vi "DAQ 다지털 실습 종합.vi"() -> ()   [LabVIEW 2020]
uses:
  <vilib>/DAQmx/read.llb/DAQmx Read (Digital 1D Bool 1Chan 1Samp).vi
  <vilib>/DAQmx/write.llb/DAQmx Write (Digital 1D Bool 1Chan 1Samp).vi
  <vilib>/DAQmx/create/channels.llb/DAQmx Create Channel (DO-Digital Output).vi
  <vilib>/DAQmx/create/channels.llb/DAQmx Create Channel (DI-Digital Input).vi
  <vilib>/DAQmx/miscellaneous.llb/DAQmx Fill In Error Info.vi
  <vilib>/DAQmx/read.llb/DAQmx Read (Digital 1D Bool NChan 1Samp 1Line).vi
panel:
  in  "정지":bool
  out "data":bool[](array[boolean]) caption="데이터"
  in  "배열":bool[](array[boolean])
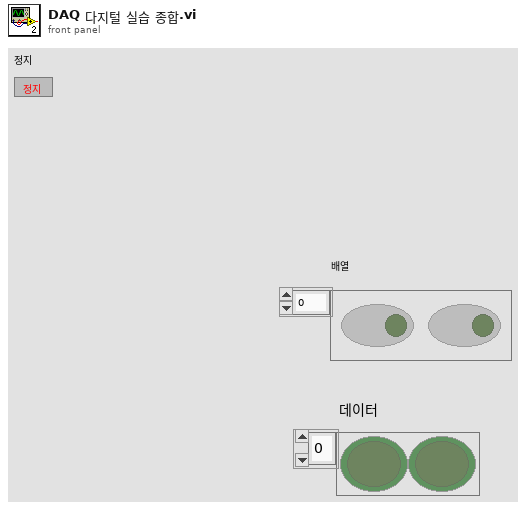
[diagram p1: front panel]
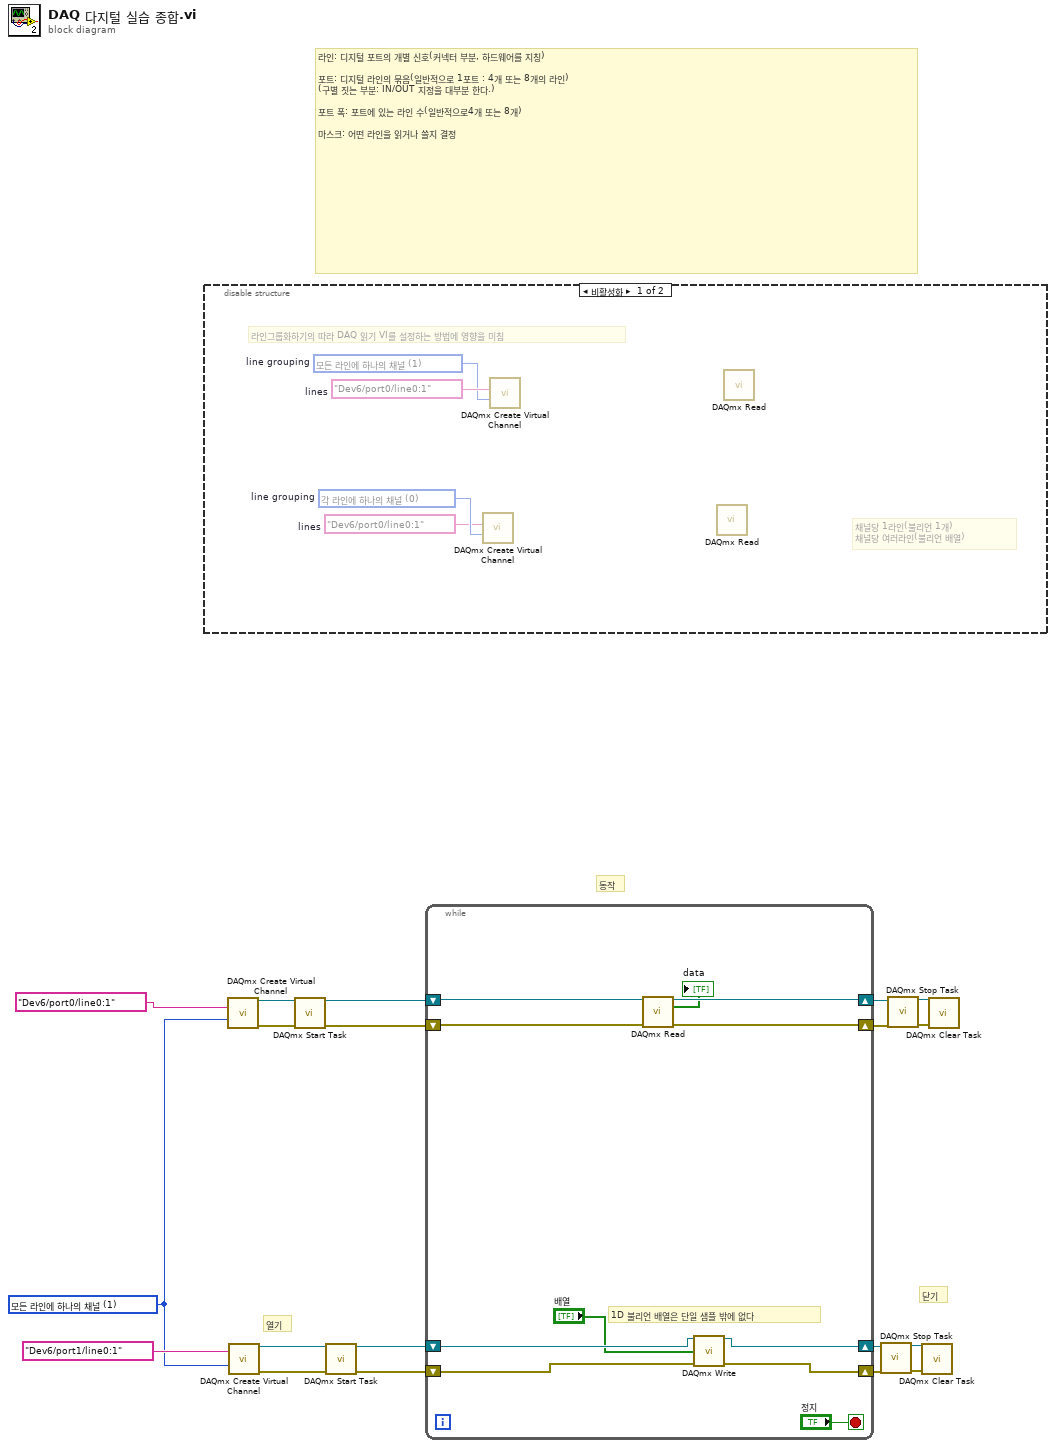
[diagram p0: block diagram]
diagram:
  w7 = 1 items=["각 라인에 하나의 채널", "모든 라인에 하나의 채널"] ("line grouping")
  # "닫기"
  # "동작"
  # "열기"
  # "라인: 디지털 포트의 개별 신호(커넥터 부분, 하드웨어를 지칭)\n\n포트: 디지털 라인의 묶음(일반적으로 1포트 : 4개 또는 8개의 라인)\n(구별 짓는 부분: IN/OUT 지정을 대부분 한다.)\n\n포트 폭: 포트에 있는 라인 수(일반적으로4개 또는 8개)\n\n마스크: 어떤 라인을 읽거나 쓸지 결정"
  n1 = disable-structure shown="비활성화" {
    frame Disabled {
      w21 = 0 items=["각 라인에 하나의 채널", "모든 라인에 하나의 채널"]  # line grouping
      w20 = tag "Dev6/port0/line0:1"  # lines
      w22 = 1 items=["각 라인에 하나의 채널", "모든 라인에 하나의 채널"]  # line grouping
      w23 = tag "Dev6/port0/line0:1"  # lines
      # "채널당 1라인(불리언 1개)\n채널당 여러라인(불리언 배열)"
      # "라인그룹화하기의 따라 DAQ 읽기 VI를 설정하는 방법에 영향을 미침"
      n2 = call-poly <vilib>:"DAQmx Create Virtual Channel.vi"("lines"=w20, "line grouping"=w21) -> ()  [unwired: 12 in, 2 out]
      n3 = call-poly <vilib>:"DAQmx Create Virtual Channel.vi"("lines"=w23, "line grouping"=w22) -> ()  [unwired: 12 in, 2 out]
      n4 = call-poly <vilib>:"DAQmx Read.vi"() -> ()  [unwired: 13 in, 3 out]
      n5 = call-poly <vilib>:"DAQmx Read.vi"() -> ()  [unwired: 13 in, 3 out]
    }
    frame Enabled {
    }
  }
  n6 = call-poly <vilib>:"DAQmx Create Virtual Channel.vi"("lines"=tag "Dev6/port0/line0:1", "line grouping"=w7) -> ("task out"=w9:refnum<k21>, "error out"=w8:errorcluster)  [unwired: 12 in]
  n7 = call-poly <vilib>:"DAQmx Create Virtual Channel.vi"("lines"=tag "Dev6/port1/line0:1", "line grouping"=w7) -> ("task out"=w18:refnum<k21>, "error out"=w17:errorcluster)  [unwired: 12 in]
  n8 = call <vilib>:"DAQmx Start Task.vi"("task/channels in"=w9, "error in"=w8) -> ("task out"=w6:refnum<k21>, "error out"=w5:errorcluster)  [unwired: 12 in]
  n9 = call <vilib>:"DAQmx Start Task.vi"("task/channels in"=w18, "error in"=w17) -> ("task out"=w16:refnum<k21>, "error out"=w15:errorcluster)  [unwired: 12 in]
  n10 = while {
    shift-right: [w32] -> w14
    shift-left: w16 -> [w34]
    shift-right: [w31] -> w13
    shift-left: w15 -> [w33]
    shift-right: [w26] -> w2
    shift-left: w6 -> [w29]
    shift-right: [w27] -> w1
    shift-left: w5 -> [w28]
    stop <- "정지" stop-if-true
    # "1D 불리언 배열은 단일 샘플 밖에 없다"
    n11 = call-poly <vilib>:"DAQmx Read.vi"("task/channels in"=w29, "error in"=w28) -> ("task out"=w26:refnum<k21>, "data"=→"data":bool[], "error out"=w27:errorcluster)  [unwired: 11 in]
    n12 = call-poly <vilib>:"DAQmx Write.vi"("task/channels in"=w34, "data"="배열", "error in"=w33) -> ("task out"=w32:refnum<k21>, "error out"=w31:errorcluster)  [unwired: 10 in, 1 out]
  }
  n13 = call <vilib>:"DAQmx Stop Task.vi"("task/channels in"=w14, "error in"=w13) -> ("task out"=w12:refnum<k21>, "error out"=w11:errorcluster)  [unwired: 12 in]
  n14 = call <vilib>:"DAQmx Stop Task.vi"("task/channels in"=w2, "error in"=w1) -> ("task out"=w3:refnum<k21>, "error out"=w4:errorcluster)  [unwired: 12 in]
  n15 = call <vilib>:"DAQmx Clear Task.vi"("task in"=w12, "error in"=w11) -> ()  [unwired: 13 in, 1 out]
  n16 = call <vilib>:"DAQmx Clear Task.vi"("task in"=w3, "error in"=w4) -> ()  [unwired: 13 in, 1 out]
